vi "CheckWidthLine(SubVI).vi"(8 "Error In":errorcluster, 11 "Input":dbl) -> (0 "Error Out":errorcluster, 3 "Output":dbl)   [LabVIEW 2018]
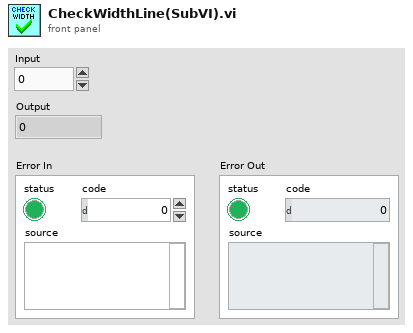
[diagram p1: front panel]
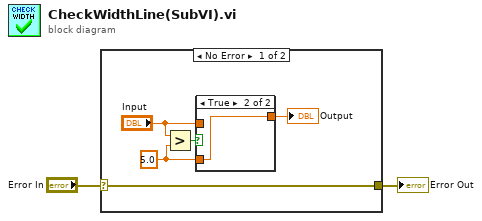
[diagram p0: block diagram]
diagram:
  n1 = case shown="No Error" "Error In" {
    selector: "Error In" -> [w3 w10]
    tunnel: [w3 w10] -> w1
    frame No Error {
      w6 = 5.0 ("y")
      n2 = Greater?(x="Input", y=w6) -> (0:w4:bool)
      n3 = case shown="True" w4 {
        tunnel: w6 -> [_ w9]
        tunnel: "Input" -> [w8 _]
        tunnel: [w8 w9] -> w7
        frame False {
        }
        frame True {
        }
      }
      "Output" <- w7
    }
    frame Error {
    }
  }
  "Error Out" <- w1
